vi "SendErrorMessageToErrorLoop.vi"(6 "Handle Loop Que":bool=TRUE, 7 "Error Message que":T1, 8 "error in (no error)":errorcluster, 11 "Loop Message que":T1) -> (0 "error out":errorcluster)   [LabVIEW 2018]
doc: "This VI forwards an error to the Error Handler Loop in a Multiple-Loop App Framework. It also tells the Error Handler Loop if the error generating loop has its que flushed, or not.\n\nThis VI needs to do the following functions:\n1. Notify Error handler\n2. Modify its own loop's execution.\n a. Abort = Flush message que and put loop in idle\nOPTIONAL, not implemted here:\n b. Pause loop, preserving the que contents, and wait for Continue/Reset/Abort loop\n i. Reset would be a special routine, like Close then Open then Start DAQ\n ii. Continue would be ignore error\n iii. Abort is the same as a., Flush message que\n\nBolder Software LLC"
uses:
  MessageQue/MessageQue.ctl
  MessageQue/MessageCluster.ctl
  MessageQue/MessageQue.lvlib
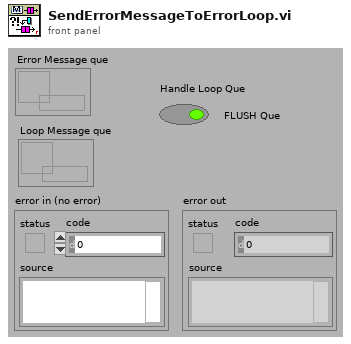
[diagram p1: front panel]
types:
  T1 = typedef "MessageQue.lvlib/MessageQue.ctl" = refnum<queue>
  T2 = cluster{"Handle Loop Que":bool, "error IO":errorcluster}
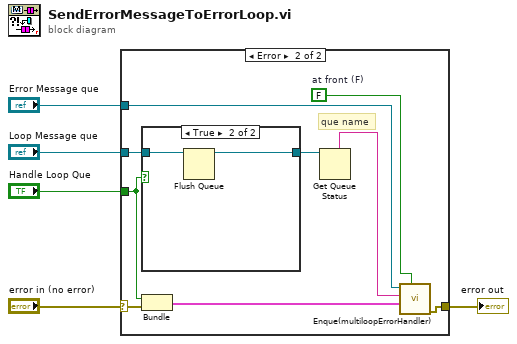
[diagram p0: block diagram]
diagram:
  n1 = case shown="Error" "error in (no error)" {
    selector: "error in (no error)" -> [w6 w14]
    tunnel: [w6 w7] -> w5
    tunnel: "Handle Loop Que" -> [_ w13]
    tunnel: "Loop Message que" -> [_ w12]
    tunnel: "Error Message que" -> [_ w11]
    frame No Error {
    }
    frame Error {
      w10 = FALSE  # at front (F)
      # "que name"
      n2 = case shown="True" w13 {
        tunnel: [w16 w17] -> w15
        tunnel: w12 -> [w16 w18]
        frame False {
          # "Could take cache action \nhere\n1. send que contents to \nthe Error Handler\n2. Drop Wait case on\ntop of local que"
        }
        frame True {
          n3 = Flush Queue(queue=w18) -> (queue out=w17:T1)  [unwired: 1 in, 2 out]
        }
      }
      n4 = Bundle("Handle Loop Que"=w13, "error IO"=w14) -> (w8:T2)  [unwired: 1 out]
      n5 = Get Queue Status(queue=w15) -> (queue name=w9:string)  [unwired: 1 in, 8 out]
      n6 = call "Enque(multiloopErrorHandler).vi"("at front (F)"=w10, "Message Payload  multiloopError cluster"=w8, "Message Command"=w9, "Message que"=w11) -> ("error out"=w7:errorcluster)  [unwired: 6 in, 1 out]
    }
  }
  "error out" <- w5
